vi "Array To Spreadsheet String.vi"(5 "Row Delimiter (;)":string="; ", 7 "Sample Delimiter (,)":string=", ", 10 "1D Array":dbl[](array[numeric]), 11 "2D Array":dbl[][](array[numeric])) -> (2 "1D Spreadsheet String":string, 3 "2D Spreadsheet String":string)   [LabVIEW 2015, in "Neural Network.lvclass"]
uses:
  Neural Network.lvclass
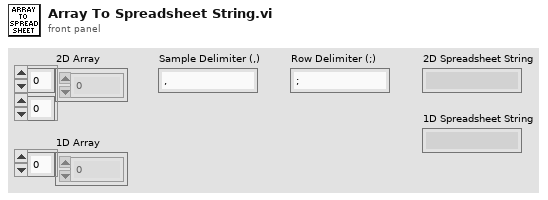
[diagram p1: front panel]
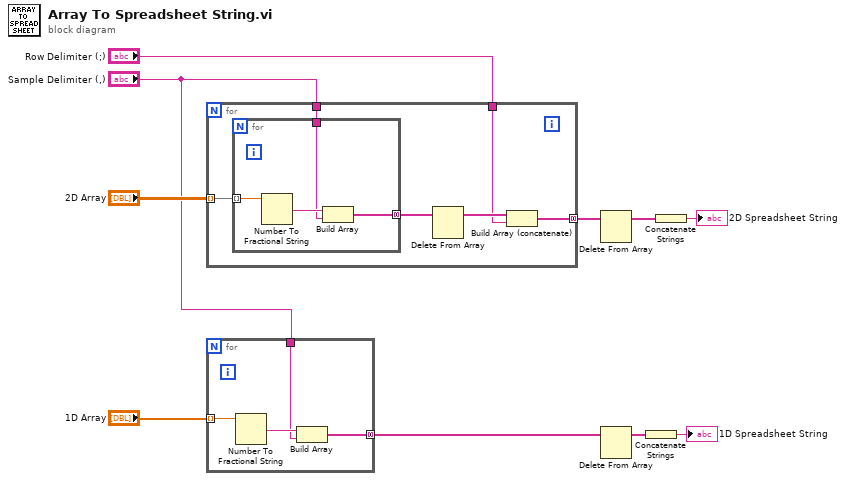
[diagram p0: block diagram]
diagram:
  n1 = for {
    tunnel: "2D Array" -> [w16] mode=indexing
    tunnel: [w15] -> w9 mode=concatenating
    tunnel: "Row Delimiter (;)" -> [w12]
    tunnel: "Sample Delimiter (,)" -> [w11]
    n2 = for {
      tunnel: w16 -> [w20] mode=indexing
      tunnel: [w18] -> w14 mode=concatenating
      tunnel: w11 -> [w17]
      n3 = Number To Fractional String(number=w20) -> (F-format string=w19:string)  [unwired: 3 in]
      n4 = Build Array(w19, w17) -> (w18:string[])
    }
    n5 = Delete From Array(array=w14) -> (array with subset deleted=w13:string[])  [unwired: 2 in, 1 out]
    n6 = Build Array (concatenate)(w13, w12) -> (w15:string[])
  }
  n7 = for {
    tunnel: "1D Array" -> [w24] mode=indexing
    tunnel: [w22] -> w2 mode=concatenating
    tunnel: "Sample Delimiter (,)" -> [w21]
    n8 = Number To Fractional String(number=w24) -> (F-format string=w23:string)  [unwired: 3 in]
    n9 = Build Array(w23, w21) -> (w22:string[])
  }
  n10 = Delete From Array(array=w9) -> (array with subset deleted=w8:string[])  [unwired: 2 in, 1 out]
  n11 = Delete From Array(array=w2) -> (array with subset deleted=w4:string[])  [unwired: 2 in, 1 out]
  n12 = Concatenate Strings(w4) -> (→"1D Spreadsheet String":string)
  n13 = Concatenate Strings(w8) -> (→"2D Spreadsheet String":string)
